vi "Generate New ID.vi"(8 "error in (no error)":errorcluster, 11 "error list in":variant) -> (0 "error out":errorcluster, 2 "new ID":string, 3 "error list out":variant)   [LabVIEW 2017]
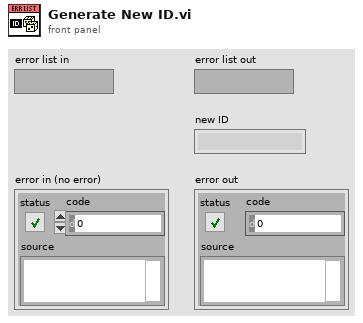
[diagram p1: front panel]
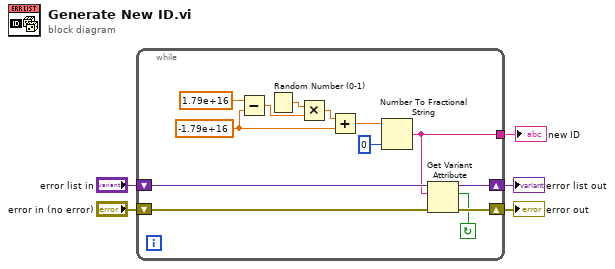
[diagram p0: block diagram]
diagram:
  n1 = while {
    shift-right: [w17] -> w2
    shift-left: "error list in" -> [w16]
    shift-right: [w15] -> w1
    shift-left: "error in (no error)" -> [w14]
    tunnel: [w6] -> w5
    stop <- w13 continue-if-true
    w8 = -1.79e+16 ("Low")
    n2 = Subtract(x=1.79e+16 ("High"), y=w8) -> (x-y=w11:dbl)
    n3 = Random Number (0-1)() -> (number: 0 to 1=w10:dbl)
    n4 = Multiply(x=w10, y=w11) -> (x*y=w12:dbl)
    n5 = Add(x=w12, y=w8) -> (x+y=w7:dbl)
    n6 = Number To Fractional String(number=w7, precision (6)=i16 0) -> (F-format string=w6:string)  [unwired: 2 in]
    n7 = Get Variant Attribute(Variant=w16, name=w6, error in=w14) -> (duplicate Variant=w17:variant, found=w13:bool, error out=w15:errorcluster)  [unwired: 1 in, 1 out]
  }
  "new ID" <- w5
  "error list out" <- w2
  "error out" <- w1
